vi "Read Sample.vi"(11 "Sample in":refnum<class "Sample.lvclass">) -> (0 "Sample In":bool, 1 "Ti Cathode":i8, 2 "Name":string, 3 "Sample out":refnum<class "Sample.lvclass">, 4 "Color":u32(colorbox))   [LabVIEW 2015, in "Sample.lvclass"]
uses:
  Sample.lvclass
  Sample.lvclass/Sample.ctl
  Controls/Ti Colors.ctl
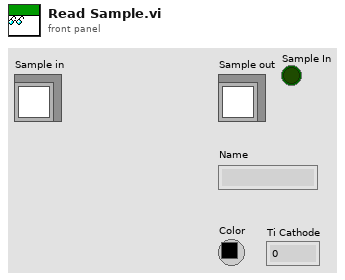
[diagram p1: front panel]
types:
  T1 = typedef "Ti Colors.ctl" = u32[]
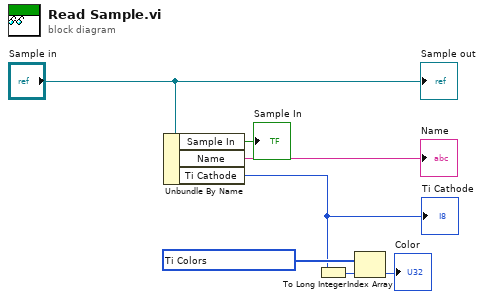
[diagram p0: block diagram]
diagram:
  n1 = Unbundle By Name("Sample in") -> ("Sample In"=→"Sample In":bool, "Name"=→"Name":string, "Ti Cathode"=w4:i8)
  "Ti Cathode" <- w4
  n2 = To Long Integer(number=w4) -> (32bit integer=w3:i32)
  n3 = Index Array(array=T1 [418898, 837796, 1256694, 1675592, 2094490, 2513388, 2932286, 3351184, 3770082, 4188980, 4607878, 5026776, 5445674, 5864572, 6283470, 6702368, 7121266, 7540164, 7959062, 8377960, 8796858, 9215756, 9634654, 10053552, 10472450, 10891348, 11310246, 11729144, 12148042, 12566940, 12985838, 13404736, 13823634, 14242532, 14661430, 15080328, 15499226, 15918124, 16337022, 16755920] ("output array 2"), index=w3) -> (element=→"Color":u32)
  "Sample out" <- "Sample in"
